vi "tcsOfc_salEvent_rejectedCommand.vi"(8 "error in (no error)":errorcluster) -> (0 "error out":errorcluster, 3 "function return":i32)   [LabVIEW 2016, in "SALLV_tcsOfc.lvlib"]
doc: "int tcsOfc_shm_salEvent_rejectedCommandLV();"
uses:
  SALLV_tcsOfc.lvlib
  SALLV_tcsOfc.so
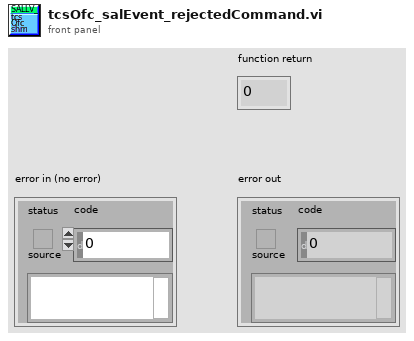
[diagram p1: front panel]
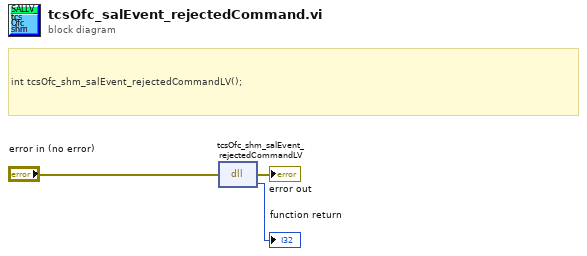
[diagram p0: block diagram]
diagram:
  # "int tcsOfc_shm_salEvent_rejectedCommandLV();"
  n1 = dll-call lib="home/ttsai/Documents/salAPI/SALLV_tcsOfc/SALLV_tcsOfc.*" fn="tcsOfc_shm_salEvent_rejectedCommandLV"(error in="error in (no error)") -> (error out=→"error out":errorcluster, →"function return":i32)  [unwired: 2 in, 1 out]
